vi "Systeminfo_Memory.vi"() -> ()   [LabVIEW 2017]
panel:
  out "array":string[][](array[string])
  out "standard output":string
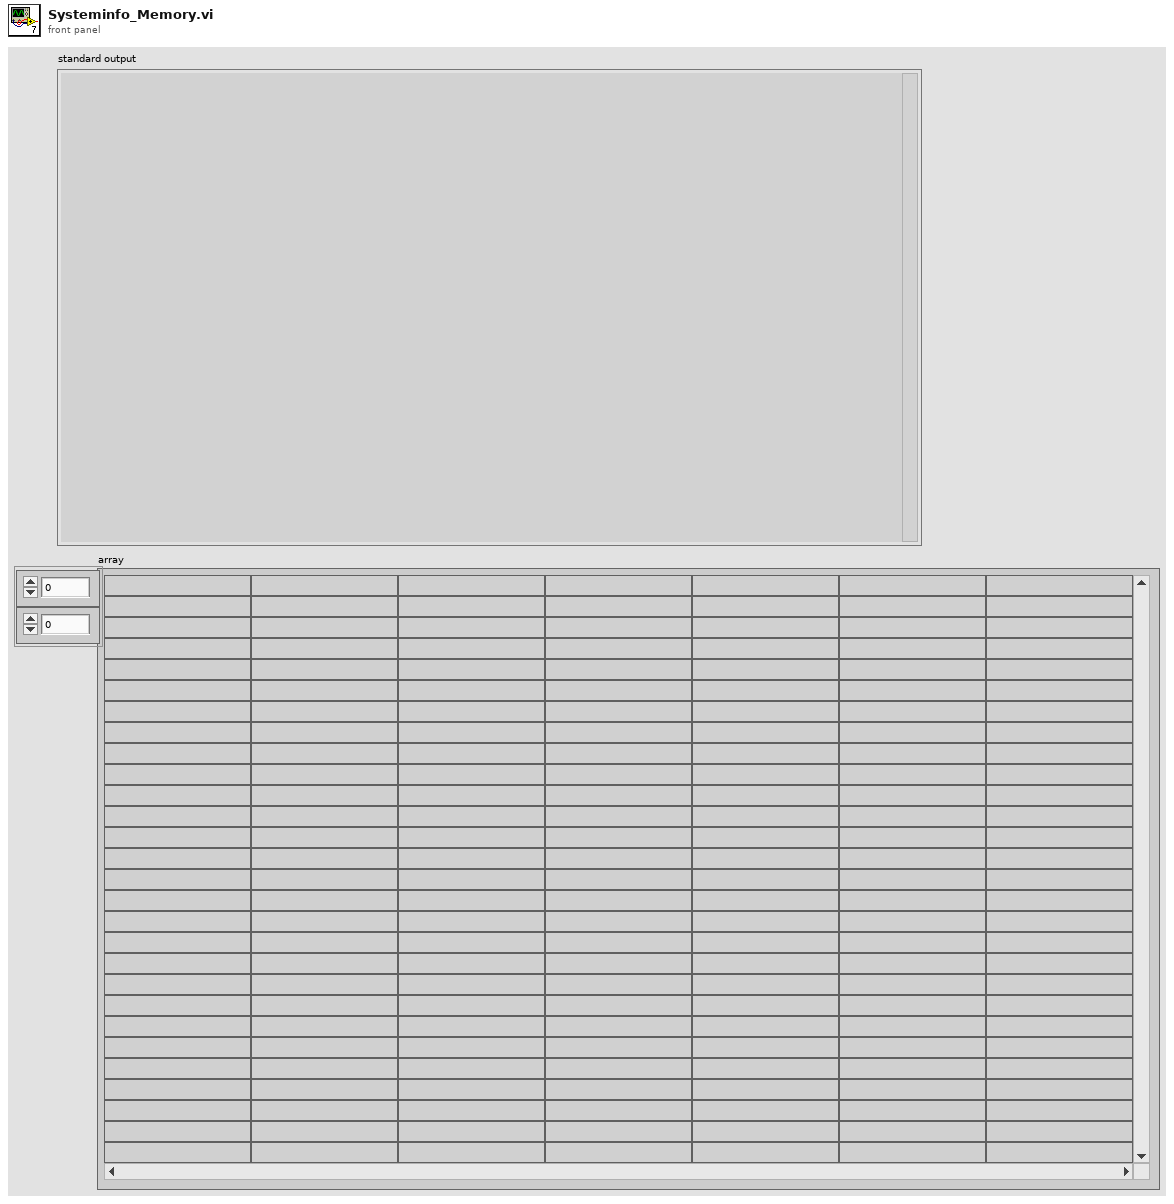
[diagram p1: front panel]
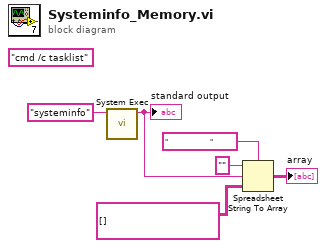
[diagram p0: block diagram]
diagram:
  (unwired) "cmd /c tasklist" ("command line")
  n1 = call <vilib>:"System Exec.vi"("command line"="systeminfo") -> ("standard output"=w3:string)  [unwired: 7 in, 3 out]
  "standard output" <- w3
  n2 = Spreadsheet String To Array(delimiter (Tab)="                     ", format string="", spreadsheet string=w3, array type (2D Dbl)=string[][] []) -> (array=→"array":string[][])
